vi "DIO_out.vi"(8 "State":bool, 9 "Digital Pin":string(combo)="Y9", 11 "Data In":T1) -> (3 "Data Out":T1={"Port"="", "All Code"="Hi"})   [LabVIEW 2016]
uses:
  uPythonX/PythonData.ctl
  uPythonX/uPythonX.xctl
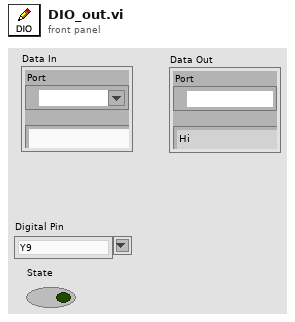
[diagram p1: front panel]
types:
  T1 = typedef "uPythonX.xctl/PythonData.ctl" = cluster{"Port":refnum<visa-resource-name>, "All Code":string}
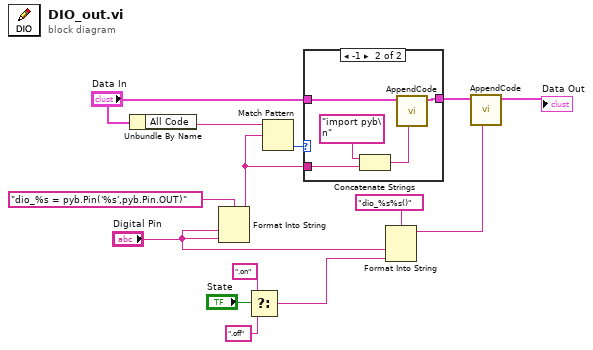
[diagram p0: block diagram]
diagram:
  n1 = Unbundle By Name("Data In") -> ("All Code"=w12:string)
  n2 = Format Into String(format string="dio_%s = pyb.Pin('%s',pyb.Pin.OUT)", "Digital Pin", "Digital Pin") -> (resulting string=w9:string)  [unwired: 2 in, 1 out]
  n3 = Select(t=".on" ("format string"), s="State", f=".off" ("format string")) -> (s? t:f=w1:string)
  n4 = Match Pattern(string=w12, regular expression=w9) -> (offset past match=w11:i32)  [unwired: 1 in, 3 out]
  n5 = case shown="-1" w11 {
    tunnel: "Data In" -> [w15 w20]
    tunnel: w9 -> [_ w17]
    tunnel: [w15 w19] -> w8
    frame Default {
    }
    frame -1 {
      n6 = Concatenate Strings("import pyb\n" ("format string"), w17) -> (w16:string)
      n7 = call "AppendCode.vi"("New Code"=w16, "Data In"=w20) -> ("Data Out"=w19:T1)  [unwired: 9 in]
    }
  }
  n8 = Format Into String(format string="dio_%s%s()", "Digital Pin", w1) -> (resulting string=w5:string)  [unwired: 2 in, 1 out]
  n9 = call "AppendCode.vi"("New Code"=w5, "Data In"=w8) -> ("Data Out"=→"Data Out":T1)  [unwired: 9 in]
